vi "Read Message.vi"(8 "Error In":errorcluster, 11 "Data In":T1) -> (0 "error out":errorcluster, 2 "number of devices":i32, 3 "Data Out":T1)   [LabVIEW 2014]
uses:
  Controls/TCP State Machine Data.ctl
  Controls/Websocket Data.ctl
  <vilib>/MediaMongrels Ltd/WebSockets/WebSockets/WebSockets.lvlib
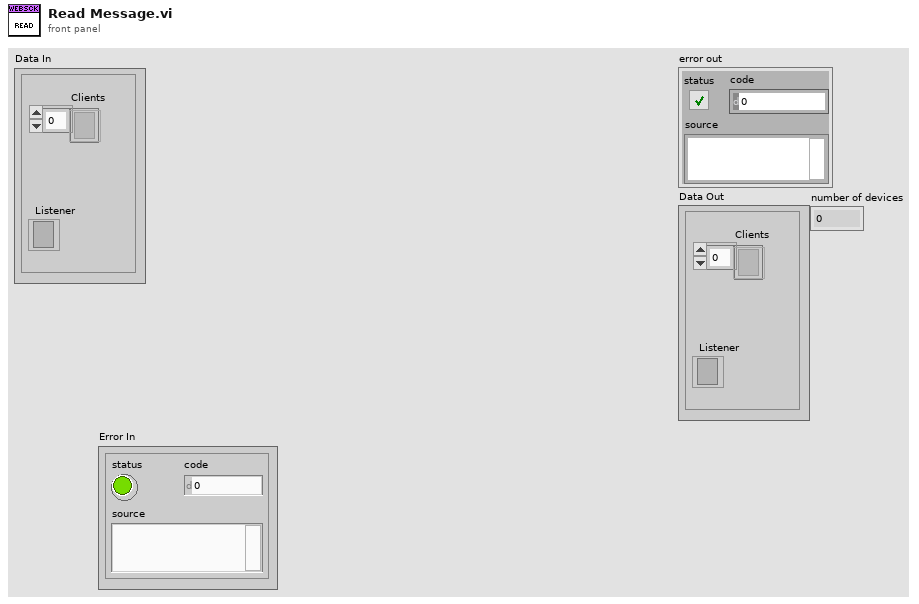
[diagram p1: front panel]
types:
  T1 = typedef "TCP State Machine Data.ctl" = cluster{"Clients":refnum<k5>[], "Listener":refnum<k5>}
  T2 = typedef "Websocket Data.ctl" = cluster{"Command":string, "Data":string}
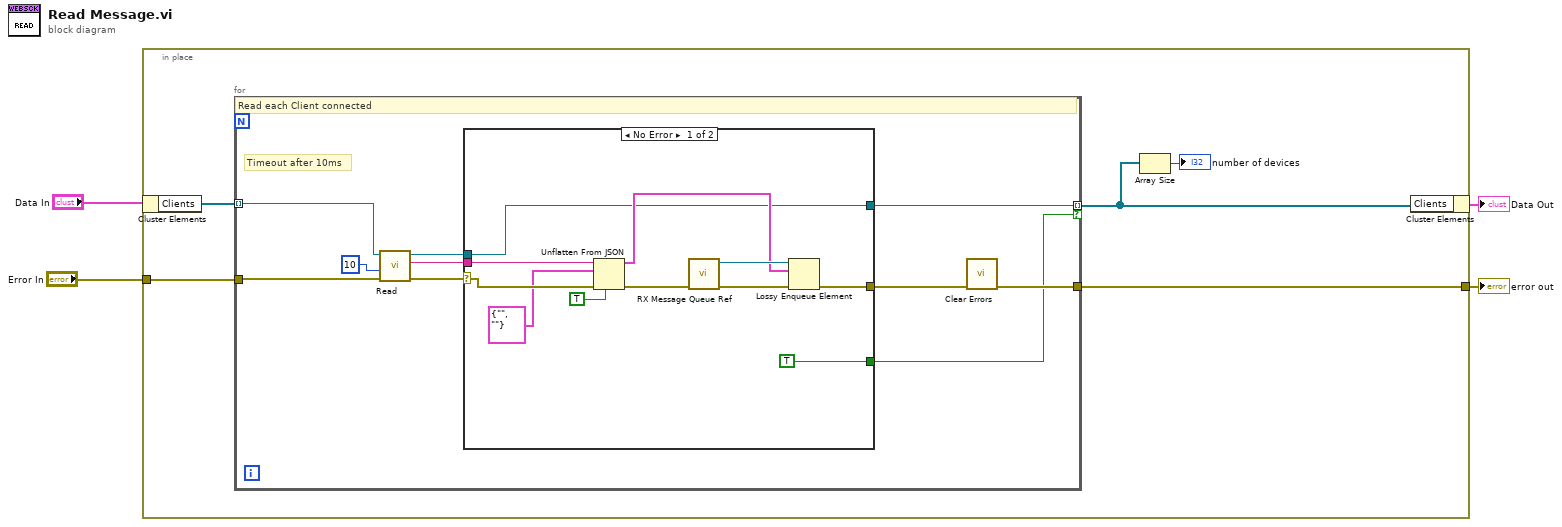
[diagram p0: block diagram]
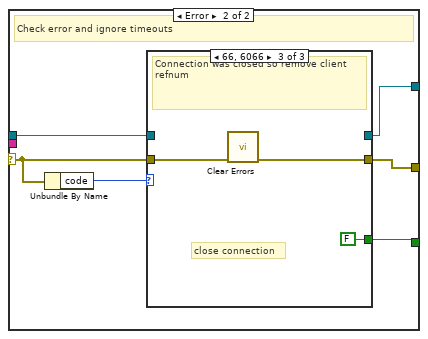
[diagram p2: hidden frame]
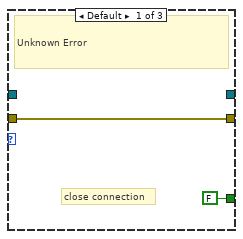
[diagram p3: hidden frame]
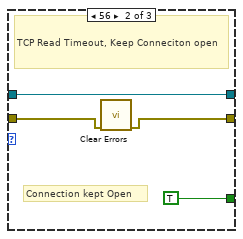
[diagram p4: hidden frame]
diagram:
  n1 = in-place {
    in-place-border: "Error In" -> [w8]
    in-place-border: [w7] -> w2
    n2 = in-place-cluster #1("Data In") -> ("Clients"=w9:refnum<k5>[])
    n3 = for {
      tunnel: w9 -> [w17] mode=indexing
      tunnel: w8 -> [w19]
      tunnel: [w12] -> w6 mode=indexing if=w10
      tunnel: [w11] -> w7
      # "Timeout after 10ms"
      # "Read each Client connected"
      n4 = call <vilib>:"Read.vi"("error in (no error)"=w19, "timeout ms (5000)"=10, "WebSocket Connection in"=w17) -> ("error out"=w16:errorcluster, "Data"=w14:string, "WebSocket Connection out"=w15:refnum<k5>)  [unwired: 5 in, 1 out]
      n5 = case shown="No Error" w16 {
        selector: w16 -> [w29 w34]
        tunnel: w15 -> [w21 w33]
        tunnel: w14 -> [w30 _]
        tunnel: [w22 w35] -> w13
        tunnel: [w21 w32] -> w12
        tunnel: [TRUE w31] -> w10
        frame No Error {
          n6 = Unflatten From JSON(JSON string=w30, type and defaults=T2 {"Command"="", "Data"=""} ("Websocket Data"), default null elements? (F)=TRUE, error in (no error)=w29) -> (value=w23:T2, error out=w26:errorcluster)  [unwired: 3 in]
          n7 = call "RX Message Queue Ref.vi"("Error In"=w26) -> ("error out"=w25:errorcluster, "rx queue ref"=w24:refnum<queue>)  [unwired: 9 in]
          n8 = Lossy Enqueue Element(queue=w24, element=w23, error in (no error)=w25) -> (error out=w22:errorcluster)  [unwired: 3 out]
        }
        frame Error {
          # "Check error and ignore timeouts"
          n9 = Unbundle By Name(w34) -> ("code"=w36:i32)
          n10 = case shown="66, 6066" w36 {
            tunnel: [w38 w41 w45] -> w35
            tunnel: w34 -> [w38 w42 w44]
            tunnel: w33 -> [_ w40 _]
            tunnel: [_ w40 _] -> w32
            tunnel: [FALSE TRUE FALSE] -> w31
            frame Default {
              # "close connection"
              # "Unknown Error"
            }
            frame 56 {
              # "Connection kept Open"
              # "TCP Read Timeout, Keep Conneciton open"
              n11 = call <vilib>:"Clear Errors.vi"("error in (no error)"=w42) -> ("error out"=w41:errorcluster)  [unwired: 5 in, 1 out]
            }
            frame 66, 6066 {
              # "close connection"
              # "Connection was closed so remove client refnum"
              n12 = call <vilib>:"Clear Errors.vi"("error in (no error)"=w44) -> ("error out"=w45:errorcluster)  [unwired: 5 in, 1 out]
            }
          }
        }
      }
      n13 = call <vilib>:"Clear Errors.vi"("error in (no error)"=w13) -> ("error out"=w11:errorcluster)  [unwired: 5 in, 1 out]
    }
    n14 = Array Size(array=w6) -> (size(s)=→"number of devices":i32)
    n15 = in-place-cluster #1("Clients"=w6) -> (→"Data Out":T1)
  }
  "error out" <- w2
